vi "saveImage.vi"(8 "error in (no error)":errorcluster, 9 "I16bit image data":u16[][](array[numeric]), 11 "Pixelfly in":refnum<class "PixelflySA.lvclass">) -> (0 "error out":errorcluster, 3 "Pixelfly out":refnum<class "PixelflySA.lvclass">)   [LabVIEW 2011, in "PixelflySA.lvclass"]
uses:
  PixelflySA.lvclass
  PixelflySA.lvclass/PixelflySA.ctl
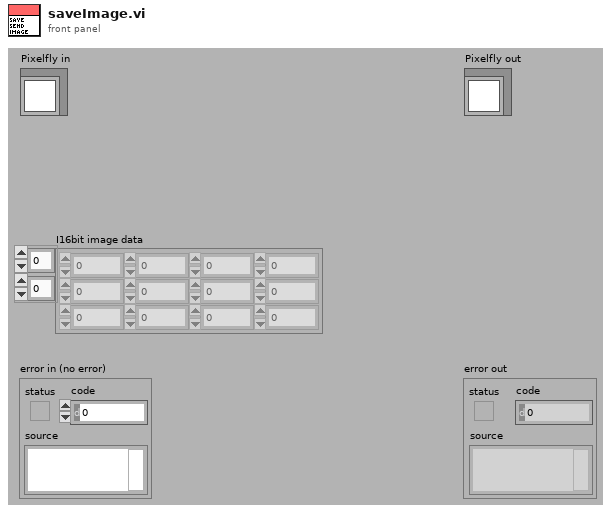
[diagram p1: front panel]
types:
  T1 = cluster{"cameraType":string, "imageName":string, "saved":string, "analysisType":string, "I16bit image data":u16[][], "path":path}
  T2 = typedef "Image Type" = u32
  T3 = typedef "IMAQ Image.ctl" = refnum<image>
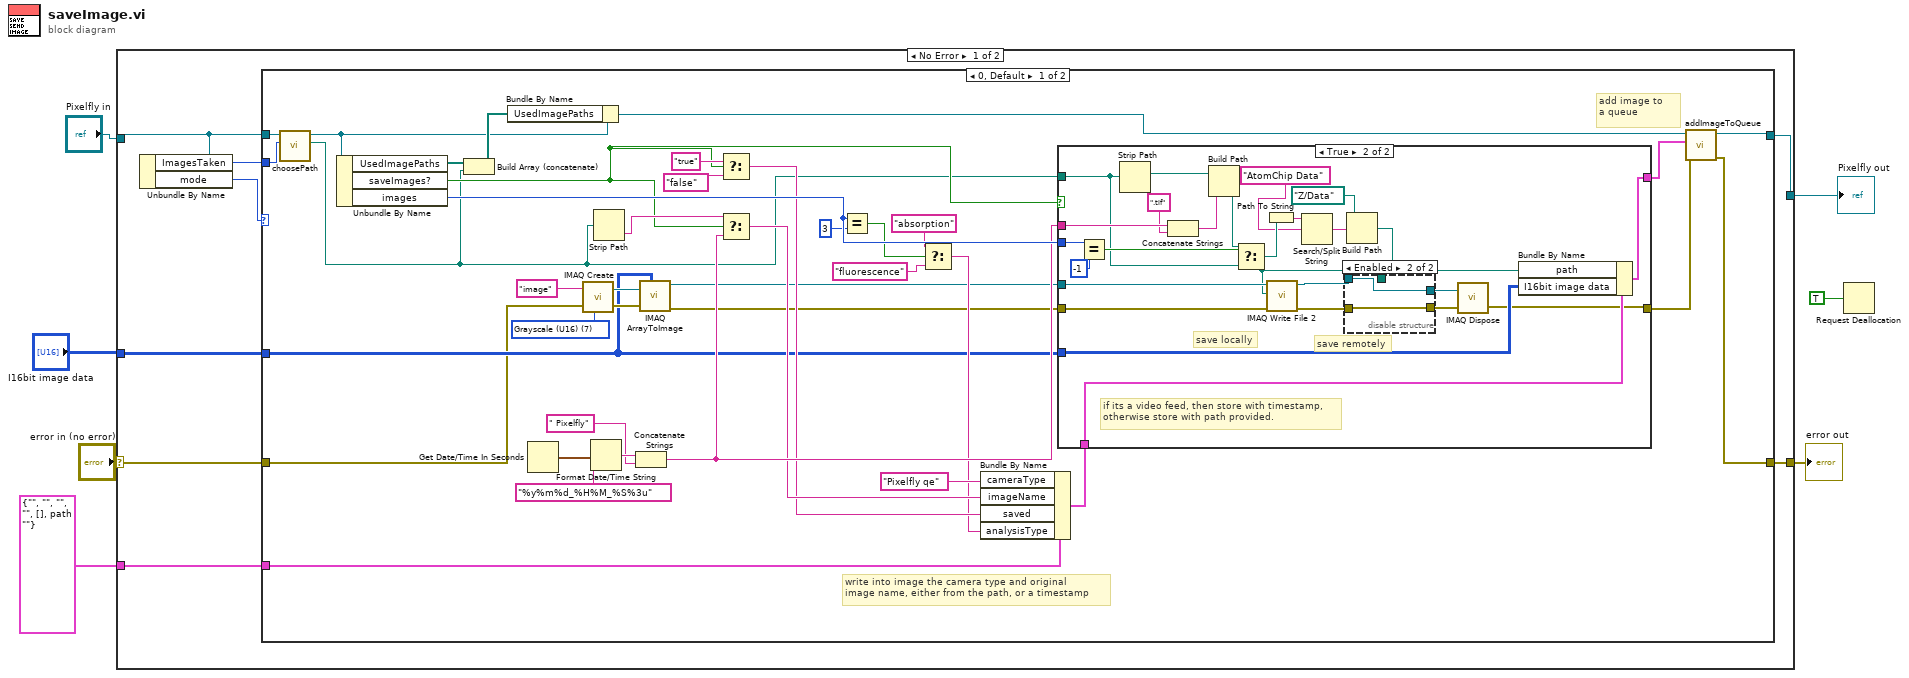
[diagram p0: block diagram]
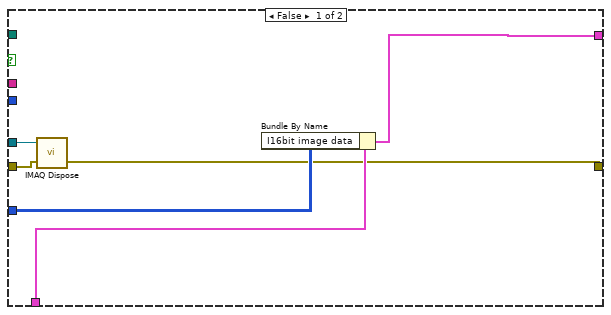
[diagram p2: hidden frame]
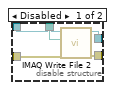
[diagram p3: hidden frame]
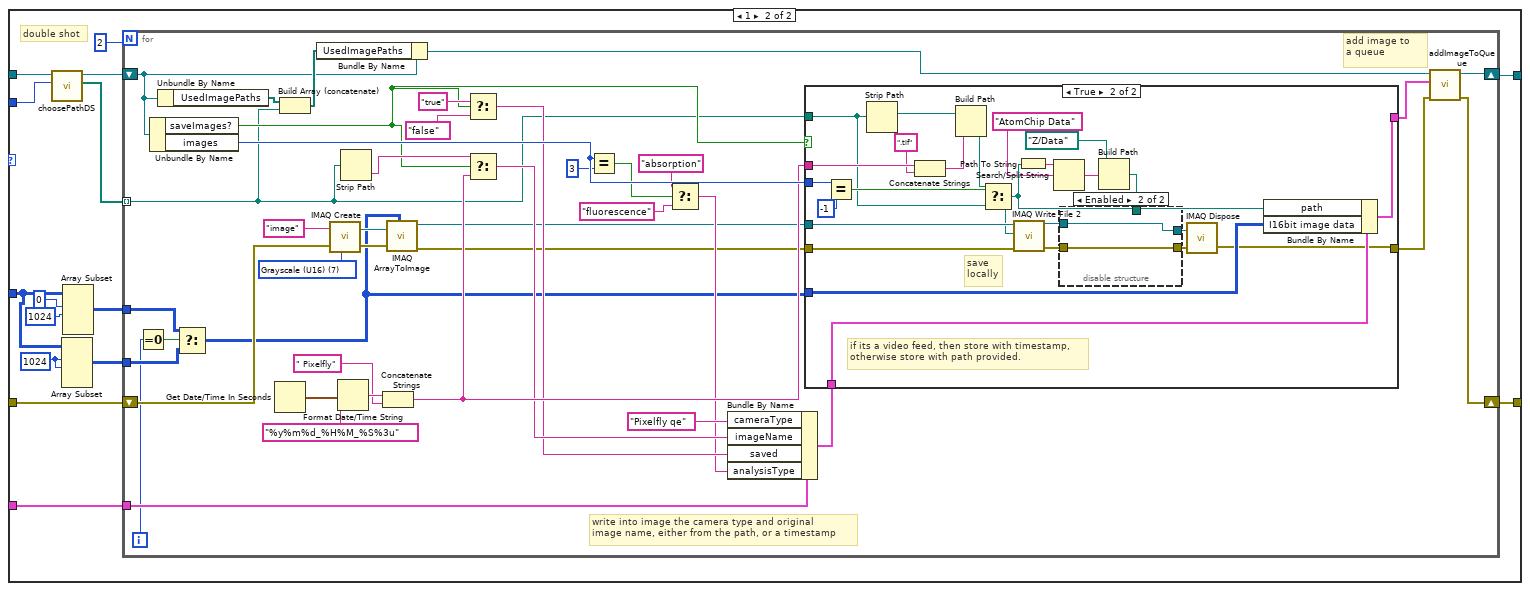
[diagram p4: hidden frame]
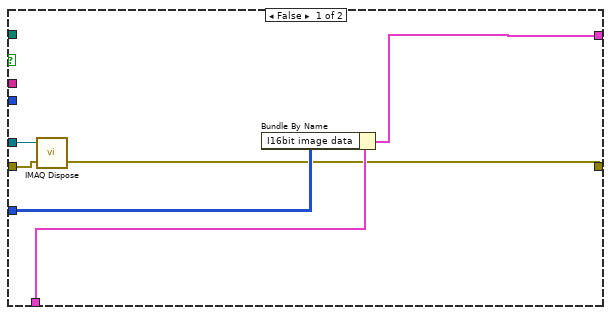
[diagram p5: hidden frame]
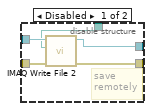
[diagram p6: hidden frame]
diagram:
  n1 = case shown="No Error" "error in (no error)" {
    selector: "error in (no error)" -> [w13 w188]
    tunnel: [w11 w188] -> w6
    tunnel: [w12 w187] -> w4
    tunnel: "Pixelfly in" -> [w10 w187]
    tunnel: "I16bit image data" -> [w14 _]
    tunnel: T1 {"cameraType"="", "imageName"="", "saved"="", "analysisType"="", "I16bit image data"=[], "path"=path ""} ("ImageData") -> [w15 _]
    frame No Error {
      n2 = Unbundle By Name(w10) -> ("ImagesTaken"=w8:i32, "mode"=w9:u16)
      n3 = case shown="0, Default" w9 {
        tunnel: w15 -> [w37 w107]
        tunnel: w14 -> [w29 w100]
        tunnel: w13 -> [w28 w106]
        tunnel: w10 -> [w22 w96]
        tunnel: [w26 w105] -> w12
        tunnel: [w23 w104] -> w11
        tunnel: w8 -> [w21 w93]
        frame 0, Default {
          w53 = T2 7 items=["Grayscale (U8)", "Grayscale (I16)", "Grayscale (SGL)", "Complex (CSG)", "RGB (U32)", "HSL (U32)", "RGB (U64)", "Grayscale (U16)"] ("Image Type")
          # "write into image the camera type and original\nimage name, either from the path, or a timestamp"
          # "add image to\na queue"
          n4 = call "choosePath.vi"("ImagesTaken"=w21, "Pixelfly in"=w22) -> ("Path"=w19:path, "Pixelfly out"=w17:refnum<class "PixelflySA.lvclass">)  [unwired: 7 in, 1 out]
          n5 = Unbundle By Name(w17) -> ("UsedImagePaths"=w20:path[], "saveImages?"=w27:bool, "images"=w44:i32)
          n6 = Build Array (concatenate)(w20, w19) -> (w18:path[])
          n7 = Bundle By Name(cluster=w17, "UsedImagePaths"=w18) -> (w16:refnum<class "PixelflySA.lvclass">)
          n8 = Get Date/Time In Seconds() -> (seconds since 1Jan1904=w50:timestamp)
          n9 = call "IMAQ Create"("Image Name"="image", "Image Type"=w53, "error in (no error)"=w28) -> ("New Image"=w52:T3, "error out"=w51:errorcluster)  [unwired: 2 in]
          n10 = Format Date/Time String(time format string (%c)="%y%m%d_%H%M_%S%3u", seconds (now)=w50) -> (date/time string=w48:string)  [unwired: 1 in]
          n11 = Strip Path(path=w19) -> (name=w39:string)  [unwired: 1 out]
          n12 = Concatenate Strings(w48, " Pixelfly") -> (w38:string)
          n13 = call "IMAQ ArrayToImage"("Image Pixels (U16)"=w29, "error in (no error)"=w51, "Image"=w52) -> ("error out"=w30:errorcluster, "Image Out"=w31:T3)  [unwired: 7 in]
          n14 = Select(t="true", s=w27, f="false") -> (s? t:f=w34:string)
          n15 = Select(t=w39, s=w27, f=w38) -> (s? t:f=w35:string)
          n16 = Equal?(x=w44, y=3) -> (x = y?=w42:bool)
          n17 = Select(t="absorption", s=w42, f="fluorescence") -> (s? t:f=w33:string)
          n18 = Bundle By Name(cluster=w37, "cameraType"="Pixelfly qe", "imageName"=w35, "saved"=w34, "analysisType"=w33) -> (w32:T1)
          n19 = case shown="True" w27 {
            tunnel: [w57 w73] -> w24
            tunnel: [w59 w75] -> w25
            tunnel: w19 -> [_ w77]
            tunnel: w38 -> [_ w84]
            tunnel: w44 -> [_ w81]
            tunnel: w32 -> [w60 w76]
            tunnel: w29 -> [w58 w74]
            tunnel: w31 -> [w56 w72]
            tunnel: w30 -> [w55 w71]
            frame False {
              n20 = call "IMAQ Dispose"("Image"=w56, "error in (no error)"=w55) -> ("error out"=w57:errorcluster)  [unwired: 4 in]
              n21 = Bundle By Name(cluster=w60, "I16bit image data"=w58) -> (w59:T1)
            }
            frame True {
              # "save remotely"
              # "save locally"
              # "if its a video feed, then store with timestamp,\notherwise store with path provided."
              n22 = Equal?(x=w81, y=-1) -> (x = y?=w78:bool)
              n23 = Strip Path(path=w77) -> (stripped path=w85:path)  [unwired: 1 out]
              n24 = Concatenate Strings(w84, ".tif") -> (w82:string)
              n25 = Build Path(base path=w85, name or relative path=w82) -> (appended path=w79:path)
              n26 = Select(t=w79, s=w78, f=w77) -> (s? t:f=w67:path)
              n27 = Path To String(path=w67) -> (string=w68:string)
              n28 = call-poly "IMAQ Write File 2"("error in (no error)"=w71, "File Path"=w67, "Image"=w72) -> ("error out"=w61:errorcluster, "Image Out (duplicate)"=w64:T3)  [unwired: 7 in]
              n29 = Search/Split String(string=w68, search string/char (-)="AtomChip Data") -> (match + rest of string=w69:string)  [unwired: 1 in, 2 out]
              n30 = Build Path(base path=path "Z:/Data", name or relative path=w69) -> (appended path=w65:path)
              n31 = disable-structure shown="Enabled" {
                disable-tunnel: w65 -> [w90 _]
                disable-tunnel: w64 -> [w89 w92]
                disable-tunnel: [w88 w92] -> w63
                disable-tunnel: [w87 w91] -> w62
                disable-tunnel: w61 -> [w86 w91]
                frame Disabled {
                  n32 = call-poly "IMAQ Write File 2"("error in (no error)"=w86, "File Path"=w90, "Image"=w89) -> ("error out"=w87:errorcluster, "Image Out (duplicate)"=w88:T3)  [unwired: 7 in]
                }
                frame Enabled {
                }
              }
              n33 = call "IMAQ Dispose"("Image"=w63, "error in (no error)"=w62) -> ("error out"=w73:errorcluster)  [unwired: 4 in]
              n34 = Bundle By Name(cluster=w76, "path"=w67, "I16bit image data"=w74) -> (w75:T1)
            }
          }
          n35 = call "addImageToQueue.vi"("error in (no error)"=w24, "ImageData"=w25, "PixelflySA in"=w16) -> ("error out"=w23:errorcluster, "PixelflySA out"=w26:refnum<class "PixelflySA.lvclass">)  [unwired: 7 in]
        }
        frame 1 {
          w102 = 1024
          # "double shot"
          n36 = call "choosePathDS.vi"("ImagesTaken"=w93, "Pixelfly in"=w96) -> ("paths"=w94:path[], "Pixelfly out"=w95:refnum<class "PixelflySA.lvclass">)  [unwired: 7 in, 1 out]
          n37 = Array Subset(array=w100, index (row)=w102, length (row)=w102) -> (w97:u16[][])  [unwired: 2 in]
          n38 = Array Subset(array=w100, index (row)=0, length (row)=1024) -> (w98:u16[][])  [unwired: 2 in]
          n39 = for {
            N: 2 -> [_]
            tunnel: w94 -> [w111] mode=indexing
            tunnel: w107 -> [w131]
            tunnel: w98 -> [w116]
            tunnel: w97 -> [w115]
            shift-right: [w121] -> w105
            shift-left: w95 -> [w109]
            shift-right: [w118] -> w104
            shift-left: w106 -> [w123]
            i -> [w113]
            w147 = T2 7 items=["Grayscale (U8)", "Grayscale (I16)", "Grayscale (SGL)", "Complex (CSG)", "RGB (U32)", "HSL (U32)", "RGB (U64)", "Grayscale (U16)"] ("Image Type")
            # "add image to\na queue"
            # "write into image the camera type and original\nimage name, either from the path, or a timestamp"
            n40 = Equal To 0?(x=w113) -> (x = 0?=w117:bool)
            n41 = Unbundle By Name(w109) -> ("saveImages?"=w122:bool, "images"=w138:i32)
            n42 = Unbundle By Name(w109) -> ("UsedImagePaths"=w112:path[])
            n43 = Select(t=w116, s=w117, f=w115) -> (s? t:f=w114:u16[][])
            n44 = Get Date/Time In Seconds() -> (seconds since 1Jan1904=w144:timestamp)
            n45 = Build Array (concatenate)(w112, w111) -> (w110:path[])
            n46 = Bundle By Name(cluster=w109, "UsedImagePaths"=w110) -> (w108:refnum<class "PixelflySA.lvclass">)
            n47 = call "IMAQ Create"("Image Name"="image", "Image Type"=w147, "error in (no error)"=w123) -> ("New Image"=w146:T3, "error out"=w145:errorcluster)  [unwired: 2 in]
            n48 = Format Date/Time String(time format string (%c)="%y%m%d_%H%M_%S%3u", seconds (now)=w144) -> (date/time string=w142:string)  [unwired: 1 in]
            n49 = Strip Path(path=w111) -> (name=w133:string)  [unwired: 1 out]
            n50 = Concatenate Strings(w142, " Pixelfly") -> (w132:string)
            n51 = call "IMAQ ArrayToImage"("Image Pixels (U16)"=w114, "error in (no error)"=w145, "Image"=w146) -> ("error out"=w124:errorcluster, "Image Out"=w125:T3)  [unwired: 7 in]
            n52 = Select(t="true", s=w122, f="false") -> (s? t:f=w128:string)
            n53 = Select(t=w133, s=w122, f=w132) -> (s? t:f=w129:string)
            n54 = Equal?(x=w138, y=3) -> (x = y?=w136:bool)
            n55 = Select(t="absorption", s=w136, f="fluorescence") -> (s? t:f=w127:string)
            n56 = Bundle By Name(cluster=w131, "cameraType"="Pixelfly qe", "imageName"=w129, "saved"=w128, "analysisType"=w127) -> (w126:T1)
            n57 = case shown="True" w122 {
              tunnel: [w151 w167] -> w119
              tunnel: [w153 w169] -> w120
              tunnel: w111 -> [_ w171]
              tunnel: w132 -> [_ w178]
              tunnel: w138 -> [_ w175]
              tunnel: w126 -> [w154 w170]
              tunnel: w114 -> [w152 w168]
              tunnel: w125 -> [w150 w166]
              tunnel: w124 -> [w149 w165]
              frame False {
                n58 = call "IMAQ Dispose"("Image"=w150, "error in (no error)"=w149) -> ("error out"=w151:errorcluster)  [unwired: 4 in]
                n59 = Bundle By Name(cluster=w154, "I16bit image data"=w152) -> (w153:T1)
              }
              frame True {
                # "save\nlocally"
                # "if its a video feed, then store with timestamp,\notherwise store with path provided."
                n60 = Equal?(x=w175, y=-1) -> (x = y?=w172:bool)
                n61 = Strip Path(path=w171) -> (stripped path=w179:path)  [unwired: 1 out]
                n62 = Concatenate Strings(w178, ".tif") -> (w176:string)
                n63 = Build Path(base path=w179, name or relative path=w176) -> (appended path=w173:path)
                n64 = Select(t=w173, s=w172, f=w171) -> (s? t:f=w157:path)
                n65 = call-poly "IMAQ Write File 2"("error in (no error)"=w165, "File Path"=w157, "Image"=w166) -> ("error out"=w162:errorcluster, "Image Out (duplicate)"=w160:T3)  [unwired: 7 in]
                n66 = Path To String(path=w157) -> (string=w156:string)
                n67 = Search/Split String(string=w156, search string/char (-)="AtomChip Data") -> (match + rest of string=w163:string)  [unwired: 1 in, 2 out]
                n68 = Build Path(base path=path "Z:/Data", name or relative path=w163) -> (appended path=w158:path)
                n69 = disable-structure shown="Enabled" {
                  disable-tunnel: w162 -> [w184 w185]
                  disable-tunnel: [w183 w185] -> w161
                  disable-tunnel: w160 -> [w182 w186]
                  disable-tunnel: [w181 w186] -> w159
                  disable-tunnel: w158 -> [w180 _]
                  frame Disabled {
                    # "save\nremotely"
                    n70 = call-poly "IMAQ Write File 2"("error in (no error)"=w184, "File Path"=w180, "Image"=w182) -> ("error out"=w183:errorcluster, "Image Out (duplicate)"=w181:T3)  [unwired: 7 in]
                  }
                  frame Enabled {
                  }
                }
                n71 = call "IMAQ Dispose"("Image"=w159, "error in (no error)"=w161) -> ("error out"=w167:errorcluster)  [unwired: 4 in]
                n72 = Bundle By Name(cluster=w170, "path"=w157, "I16bit image data"=w168) -> (w169:T1)
              }
            }
            n73 = call "addImageToQueue.vi"("error in (no error)"=w119, "ImageData"=w120, "PixelflySA in"=w108) -> ("error out"=w118:errorcluster, "PixelflySA out"=w121:refnum<class "PixelflySA.lvclass">)  [unwired: 7 in]
          }
        }
      }
    }
    frame Error {
    }
  }
  "error out" <- w6
  "Pixelfly out" <- w4
  n74 = Request Deallocation(TRUE ("flag")) -> ()
